vi "testParseStateQueueSimple.vi"(8 "error in (no error)":errorcluster, 11 "testStateMachineUtilities in":refnum<class "testStateMachineUtilities.lvclass">) -> (0 "error out":errorcluster, 3 "testStateMachineUtilities out":refnum<class "testStateMachineUtilities.lvclass">)   [LabVIEW 2013, in "testStateMachineUtilities.lvclass"]
uses:
  testStateMachineUtilities.lvclass
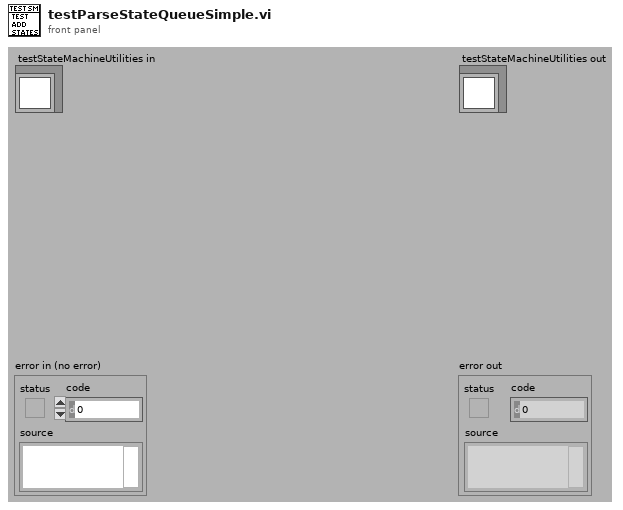
[diagram p1: front panel]
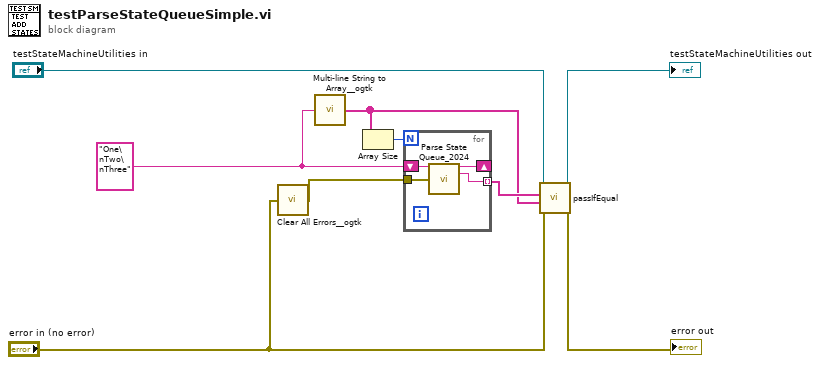
[diagram p0: block diagram]
diagram:
  w4 = "One\nTwo\nThree" ("State Queue")
  n1 = call <userlib>:"Clear All Errors__ogtk.vi"("Error In"="error in (no error)") -> ("Error Out"=w5:errorcluster)  [unwired: 3 in]
  n2 = call <userlib>:"Multi-line String to Array__ogtk.vi"("string"=w4) -> ("lines"=w1:string[])
  n3 = Array Size(array=w1) -> (size(s)=w2:i32)
  n4 = for {
    N: w2 -> [_]
    tunnel: w5 -> [w12]
    tunnel: [w11] -> w3 mode=indexing
    shift-right: [w10] -> _
    shift-left: w4 -> [w13]
    n5 = call "Parse State Queue_2024.vi"("State Queue"=w13, "Error In (no error)"=w12) -> ("Remaining States"=w10:string, "Current State"=w11:string)  [unwired: 11 in, 1 out]
  }
  n6 = call-dynamic "passIfEqual.vi"("error in (no error)"="error in (no error)", "y"=w1, "x"=w3, "TestCase in"="testStateMachineUtilities in") -> ("error out"=→"error out":errorcluster, "TestCase out"=→"testStateMachineUtilities out":refnum<class "testStateMachineUtilities.lvclass">)  [unwired: 6 in]
